vi "Update Histogram Window Menu Checks.vi"(8 "Error In":errorcluster, 9 "menu reference":refnum<k9>, 11 "XYGraph in":refnum<vi>) -> (0 "Error Out":errorcluster)   [LabVIEW 2021, in "Histogram Window.lvlib"]
uses:
  Histogram Window.lvlib
  Graphs/XY Graph/XY Graph Add-Ons.lvlib
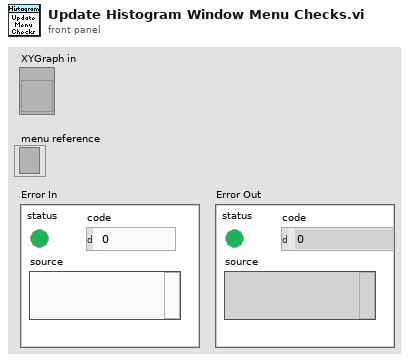
[diagram p1: front panel]
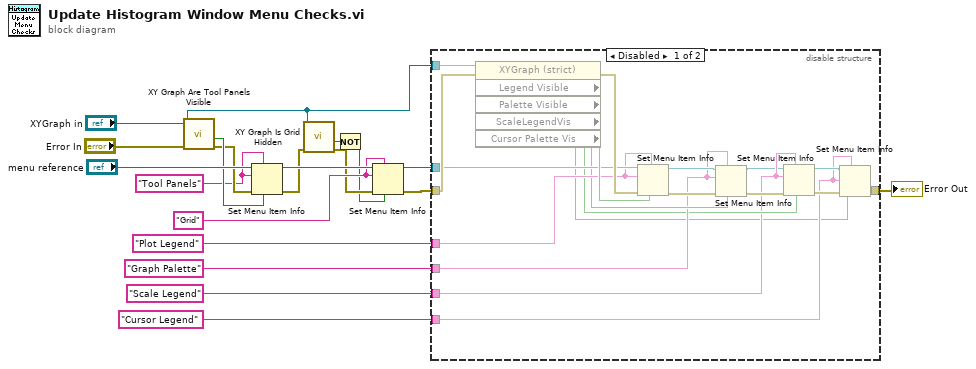
[diagram p0: block diagram]
diagram:
  w13 = "Grid" ("item name")
  w16 = "Tool Panels" ("item name")
  n1 = call "XY Graph Are Tool Panels Visible.vi"("Error In"="Error In", "XY Graph Ref"="XYGraph in") -> ("Error Out"=w17:errorcluster, "Any Panel Visible?"=w18:bool)  [unwired: 6 in, 2 out]
  n2 = Set Menu Item Info(6:w18, 7:w16, 8:w17, 10:w16, 11:"menu reference") -> (0:w5:errorcluster, 3:w14:refnum<k9>)  [unwired: 2 in]
  n3 = call "XY Graph Is Grid Hidden.vi"("Error In"=w5, "XY Graph Ref"="XYGraph in") -> ("Error Out (dup)"=w4:errorcluster, "Hidden Grid(s)"=w3:bool)  [unwired: 7 in, 1 out]
  n4 = Not(x=w3) -> (.not. x?=w2:bool)
  n5 = Set Menu Item Info(6:w2, 7:w13, 8:w4, 10:w13, 11:w14) -> (0:w12:errorcluster, 3:w11:refnum<k9>)  [unwired: 2 in]
  n6 = disable-structure shown="Disabled" {
    disable-tunnel: w12 -> [w38 w39]
    disable-tunnel: w11 -> [w35 _]
    disable-tunnel: "Plot Legend" ("item name") -> [w34 _]
    disable-tunnel: "Graph Palette" ("item name") -> [w30 _]
    disable-tunnel: "Scale Legend" ("item name") -> [w27 _]
    disable-tunnel: "Cursor Legend" ("item name") -> [w23 _]
    disable-tunnel: [w21 w39] -> w6
    disable-tunnel: "XYGraph in" -> [w20 _]
    frame Disabled {
      n7 = property class="XYGraph (strict)"(reference=w20, error in=w38) -> (error out=w36:errorcluster, "Legend Visible"=w37:bool, "Palette Visible"=w31:bool, "ScaleLegendVis"=w28:bool, "Cursor Palette Vis"=w22:bool)  [unwired: 1 out]
      n8 = Set Menu Item Info(6:w37, 7:w34, 8:w36, 10:w34, 11:w35) -> (0:w33:errorcluster, 3:w32:refnum<k9>)  [unwired: 2 in]
      n9 = Set Menu Item Info(6:w31, 7:w30, 8:w33, 10:w30, 11:w32) -> (0:w29:errorcluster, 3:w24:refnum<k9>)  [unwired: 2 in]
      n10 = Set Menu Item Info(6:w28, 7:w27, 8:w29, 10:w27, 11:w24) -> (0:w26:errorcluster, 3:w25:refnum<k9>)  [unwired: 2 in]
      n11 = Set Menu Item Info(6:w22, 7:w23, 8:w26, 10:w23, 11:w25) -> (0:w21:errorcluster)  [unwired: 2 in, 1 out]
    }
    frame Enabled {
    }
  }
  "Error Out" <- w6
